vi "Get State.vi"(8 "error in (no error)":errorcluster, 11 "TCP Comm In":T2) -> (0 "error out":errorcluster, 2 "State":T1)   [LabVIEW 2020, in "TCP Comms.lvlib"]
uses:
  TCP Comms.lvlib
  TCP Comm.ctl
  Ref Data.ctl
  State.ctl
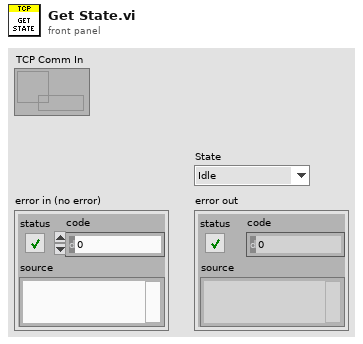
[diagram p1: front panel]
types:
  T1 = typedef "TCP Comms.lvlib/State.ctl" = enum16{"Idle", "Starting", "Connecting", "Connected", "Disconnecting", "Stopped"}
  T2 = typedef "TCP Comms.lvlib/TCP Comm.ctl" = refnum<data-value>
  T3 = typedef "TCP Comms.lvlib/Ref Data.ctl" = cluster{"TCP":refnum<k5>, "State":T1, "Server":bool, "Host":string, "Port":u16, "Listener":refnum<k5>, "Start":bool, "Disconnect":bool, "TCP Valid":bool, "TLS Enabled":bool, "Immutable TLS":refnum<k36>, "Certificate DN":string}
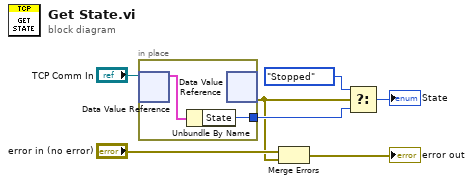
[diagram p0: block diagram]
diagram:
  n1 = in-place {
    in-place-border: [w8] -> w4
    n2 = in-place-dvr #1("TCP Comm In") -> (w9:T3)  [unwired: 1 out]
    n3 = Unbundle By Name(w9) -> ("State"=w8:T1)
    n4 = in-place-dvr #1() -> (w1:errorcluster)  [unwired: 1 in, 1 out]
  }
  n5 = Merge Errors("error in (no error)", w1) -> (→"error out":errorcluster)
  n6 = Select(t=State."Stopped", s=w1, f=w4) -> (s? t:f=→"State":T1)
